vi "Untitled 27.vi"() -> ()   [LabVIEW 2020]
uses:
  Type Descriptor Enumeration.ctl
  variant.lvclass/variant.ctl
  Type Descriptor/TD.lvclass/TD.ctl
  Bytes/Bytes.lvclass/Bytes.ctl
  Type Descriptor/get_type_enum.vi
  Bytes/read.vi
  Bytes/to_data.vi
  Bytes/from_byte_array.vi
  Type Descriptor/TD.lvclass
  C:/projects/OpenG-Variant-Data-Library/source/library/Bytes/Bytes.lvclass
  Get Data Name from TD.vi
  Bytes/Bytes.lvclass
  variant.lvclass
  openg_variant.lvlib
panel:
  out "Data out":variant
  out "error out":errorcluster
  out "Array 2":variant[](array[variant])
  out "Array":T2(array[cluster]) {"Type Descriptor Enumeration" format="%.0x"}
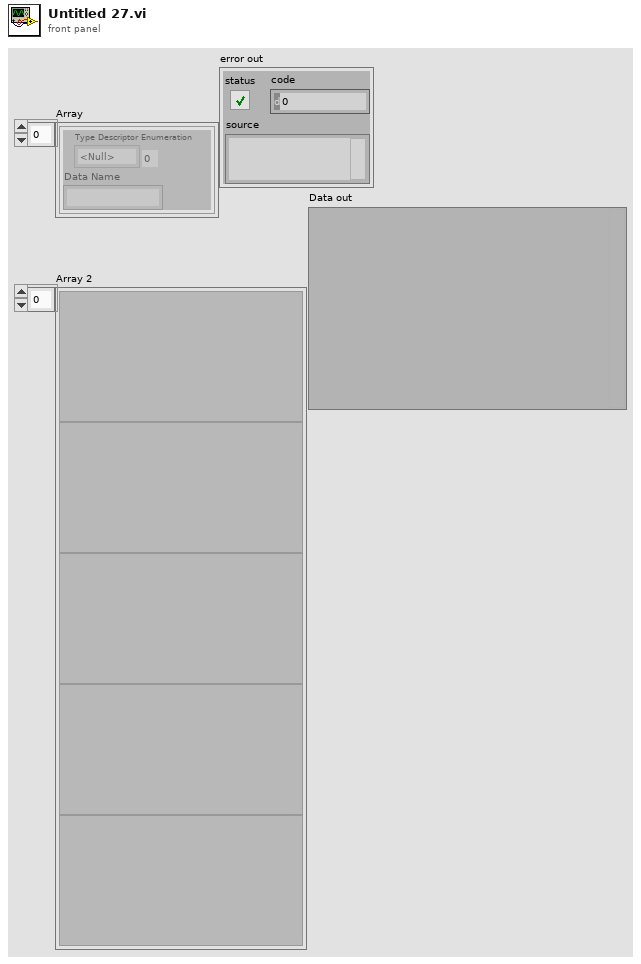
[diagram p1: front panel]
types:
  T1 = typedef "openg_variant.lvlib/Type Descriptor Enumeration.ctl" = enum8{"<Null>", "I8", "I16", "I32", "I64", "U8", "U16", "U32", "U64", "SGL", "DBL", "EXT", "CSG", "CDB", "CXT", "0x0F", "0x10", "0x11", "0x12", "0x13", "0x14", "Enum U8", "Enum U16", "Enum U32", "Enum U64", "SGL PQ", "DBL PQ", "EXT PQ", "CSG PQ", "CDB PQ", "CXT PQ", "0x1F", "0x20", "Boolean", "0x22", "0x23", "0x24", "0x25", "0x26", "0x27", "0x28", "0x29", "0x2A", "0x2B", "0x2C", "0x2D", "0x2E", "0x2F", "String", "0x31", "Path", "Pict", "0x34", "0x35", "0x36", "DAQ", "0x38", "0x39", "0x3A", "0x3B", "0x3C", "0x3D", "0x3E", "0x3F", "Array", "0x41", "0x42", "0x43", "0x44", "0x45", "0x46", "0x47", "0x48", "0x49", "0x4A", "0x4B", "0x4C", "0x4D", "0x4E", "0x4F", "Cluster", "0x51", "0x52", "Variant", "Waveform", "0x55", "0x56", "0x57", "0x58", "0x59", "0x5A", "0x5B", "0x5C", "0x5D", "0x5E", "Fixed Point", "0x60", "0x61", "0x62", "0x63", "0x64", "0x65", "0x66", "0x67", "0x68", "0x69", "0x6A", "0x6B", "0x6C", "0x6D", "0x6E", "0x6F", "Refnum", "0x71", "0x72", "Set Collection", "Map Collection"}
  T2 = cluster{"Type Descriptor Enumeration":T1, "Data Name":string}[]
  T3 = cluster{"Type Descriptor Enumeration":T1, "Data Name":string}
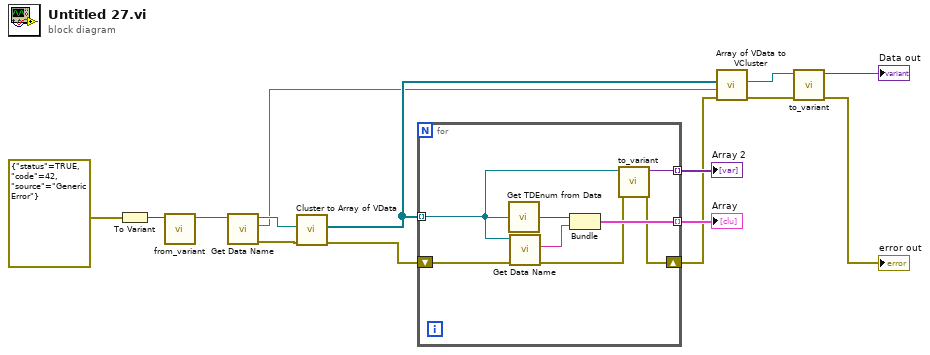
[diagram p0: block diagram]
diagram:
  n1 = To Variant(anything=errorcluster {"status"=TRUE, "code"=42, "source"="Generic Error"} ("error constant")) -> (Variant=w14:variant)
  n2 = call "from_variant.vi"("Data"=w14) -> ("LVData out"=w9:refnum<class "variant.lvclass">)  [unwired: 9 in, 1 out]
  n3 = call "Get Data Name.vi"("Data"=w9) -> ("error out"=w7:errorcluster, "Data Name"=w6:string, "Data dup"=w8:refnum<class "variant.lvclass">)  [unwired: 8 in]
  n4 = call "Cluster to Array of VData.vi"("error in (no error)"=w7, "Cluster"=w8) -> ("error out"=w11:errorcluster, "Array of VData"=w10:refnum<class "variant.lvclass">[])  [unwired: 8 in]
  n5 = for {
    tunnel: w10 -> [w20] mode=indexing
    tunnel: [w21] -> w13 mode=indexing
    tunnel: [w19] -> w12 mode=indexing
    shift-right: [w16] -> w2
    shift-left: w11 -> [w18]
    n6 = call "Get TDEnum from Data.vi"("Data"=w20) -> ("Type Descriptor Enumeration"=w23:T1)  [unwired: 4 in]
    n7 = call "Get Data Name.vi"("error in"=w18, "Data"=w20) -> ("error out"=w17:errorcluster, "Data Name"=w22:string)  [unwired: 7 in, 1 out]
    n8 = Bundle("Type Descriptor Enumeration"=w23, "Data Name"=w22) -> (w21:T3)  [unwired: 1 in]
    n9 = call "to_variant.vi"("error in (no error)"=w17, "LVData in"=w20) -> ("error out"=w16:errorcluster, "Data out"=w19:variant)  [unwired: 8 in]
  }
  "Array" <- w13
  "Array 2" <- w12
  n10 = call "Array of VData to VCluster.vi"("error in (no error)"=w2, "Cluster Name"=w6, "Array"=w10) -> ("error out"=w3:errorcluster, "VCluster"=w5:refnum<class "variant.lvclass">)  [unwired: 7 in]
  n11 = call "to_variant.vi"("error in (no error)"=w3, "LVData in"=w5) -> ("error out"=→"error out":errorcluster, "Data out"=→"Data out":variant)  [unwired: 8 in]
